vi "passTest.vi"(11 "IA state":T2={"our_robots"=[], "enemy_robots"=[], "balls"=[], "geometry"={"line_width"=0, "field_length"=0, "field_width"=0, "boundary_width"=0, "referee_width"=0, "goal_width"=0, "goal_depth"=0, "goal_wall_width"=0, "center_circle_radius"=0, "defense_radius"=0, "defense_stretch"=0, "free_kick_from_defense_dist"=0, "penalty_spot_from_field_line_dist"=0, "penalty_line_from_spot_dist"=0}, "IA Judge"={"stage"="", "command"="", "our_goalie_id"=0.0, "enemy_goalie_id"=0.0, "command enum"=enum."Halt", "Time"=enum."Azul"}, "Received Timestamp"=timestamp(0 s since 1904-01-01), "Events"={"Touch"=FALSE, "Ball out"=FALSE, "id touch"=0.0, "Ball out of \nVision"=FALSE, "Ball inside \nGoalie area"=FALSE, "Robot not responding"=FALSE, "Robots responding status"=[1.0, 1.0, 1.0, 1.0, 1.0, 1.0], "Enemy Ball \nPossession"=FALSE, "Pass State"=FALSE, "id end of pass"=0.0, "Kick"=FALSE, "Id ini Possession"=0.0, "Ball Possesion"=FALSE, "Id Possesion"=0.0}}) -> (0 "ID Kicker Robot":u32, 1 "Pass finished":bool=TRUE, 2 "ID Receiving Robot":dbl, 3 "Pass state":T1)   [LabVIEW 2017]
uses:
  Core/AI Input.ctl
  Core/AI Robot.ctl
  Intel/Functions Enum.ctl
  Intel/AttackerStates.ctl
  Core/AI Ball.ctl
  Core/Field Size.ctl
  Core/AI Judge.ctl
  Intel/Command Enum.ctl
  Util/Events/Events.ctl
  passTestStates.ctl
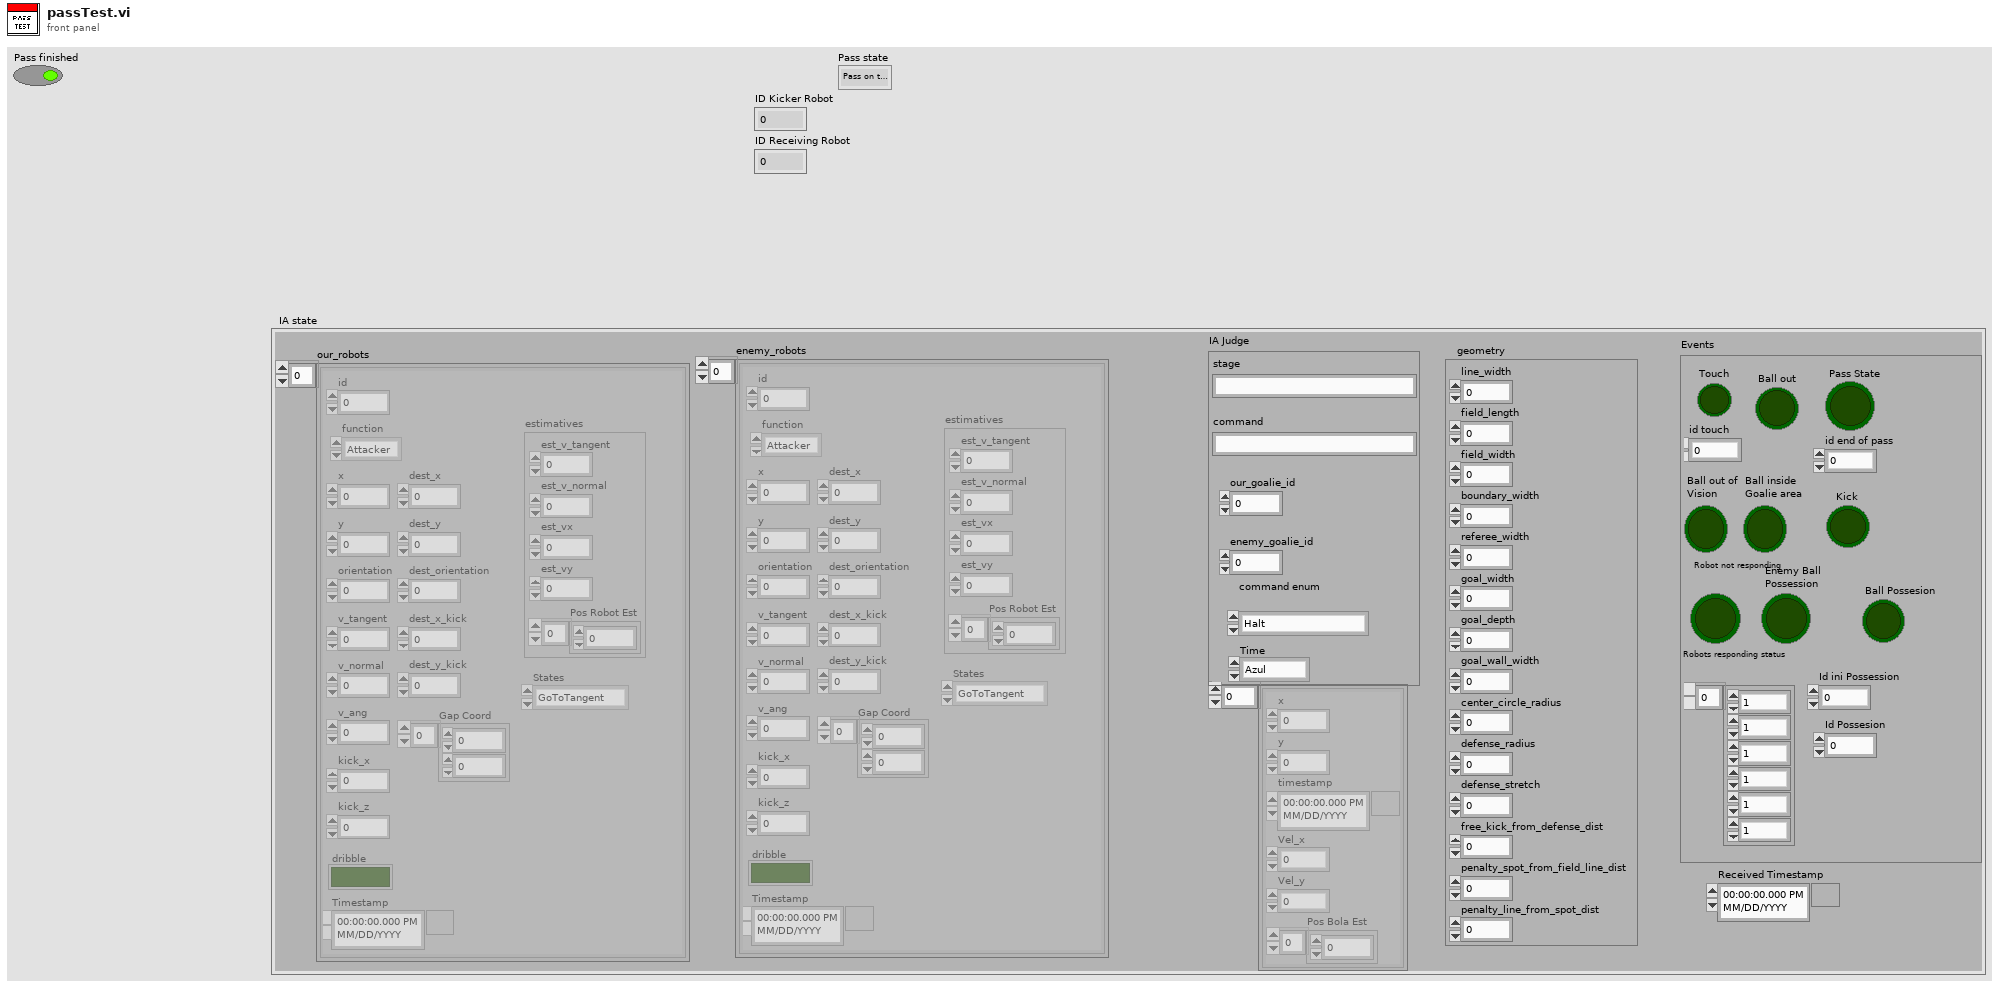
[diagram p1: front panel]
types:
  T1 = typedef "passTestStates.ctl" = enum16{"Pass on the way", "Ball stops", "Pass intercepted", "Ball out of the field", "Ball missed robot", "Need more force to pass", "Too much force", "Correct pass"}
  T2 = typedef "AI Input.ctl" = cluster{"our_robots":T3[], "enemy_robots":T3[], "balls":T6[], "geometry":T7, "IA Judge":T8, "Received Timestamp":timestamp, "Events":T10}
  T3 = typedef "AI Robot.ctl" = cluster{"id":u32, "function":T4, "x":dbl, "y":dbl, "orientation":dbl, "v_tangent":dbl, "v_normal":dbl, "v_ang":dbl, "kick_x":dbl, "kick_z":dbl, "dribble":bool, "Timestamp":timestamp, "dest_x":dbl, "dest_y":dbl, "dest_orientation":dbl, "estimatives":cluster{"est_v_tangent":dbl, "est_v_normal":dbl, "est_vx":dbl, "est_vy":dbl, "Pos Robot Est":dbl[]}, "dest_x_kick":dbl, "dest_y_kick":dbl, "Gap Coord":dbl[], "States":T5}
  T4 = typedef "Functions Enum.ctl" = enum16{"Attacker", "Goalie", "Defender", "Striker", "Goto 0", "Dummy", "Kicker", "ZigZag"}
  T5 = typedef "AttackerStates.ctl" = enum16{"Pass", "GoToTangent", "BallGetting", "GoToKick", ""}
  T6 = typedef "AI Ball.ctl" = cluster{"x":dbl, "y":dbl, "timestamp":timestamp, "Vel_x":dbl, "Vel_y":dbl, "Pos Bola Est":dbl[]}
  T7 = typedef "Field Size.ctl" = cluster{"line_width":u32, "field_length":u32, "field_width":u32, "boundary_width":u32, "referee_width":u32, "goal_width":u32, "goal_depth":u32, "goal_wall_width":u32, "center_circle_radius":u32, "defense_radius":u32, "defense_stretch":u32, "free_kick_from_defense_dist":u32, "penalty_spot_from_field_line_dist":u32, "penalty_line_from_spot_dist":u32}
  T8 = typedef "AI Judge.ctl" = cluster{"stage":string, "command":string, "our_goalie_id":dbl, "enemy_goalie_id":dbl, "command enum":T9, "Time":enum16{"Azul", "Amarelo"}}
  T9 = typedef "Command Enum.ctl" = enum16{"Halt", "Stop", "Force Start", "PKA Normal Start", "Prepare Kickoff Ally", "PKE Normal Start", "Prepare Kickoff Enemy", "Prepare Penalty Ally", "PPA Normal Start", "Prepare Penalty Enemy", "PPE Normal Start", "Direct Free Enemy", "Direct Free Ally", "Indirect Free Enemy", "Indirect Free Ally", "Timeout Enemy", "Timeout Ally", "Goal Enemy", "Goal Ally", "Ball Placement Enemy", "Ball Placement Ally", "Normal Half Time", "Extra Time Break", "Extra Half Time", "None", "Post Game"}
  T10 = typedef "Events.ctl" = cluster{"Touch":bool, "Ball out":bool, "id touch":dbl, "Ball out of \nVision":bool, "Ball inside \nGoalie area":bool, "Robot not responding":bool, "Robots responding status":dbl[], "Enemy Ball \nPossession":bool, "Pass State":bool, "id end of pass":dbl, "Kick":bool, "Id ini Possession":dbl, "Ball Possesion":bool, "Id Possesion":dbl}
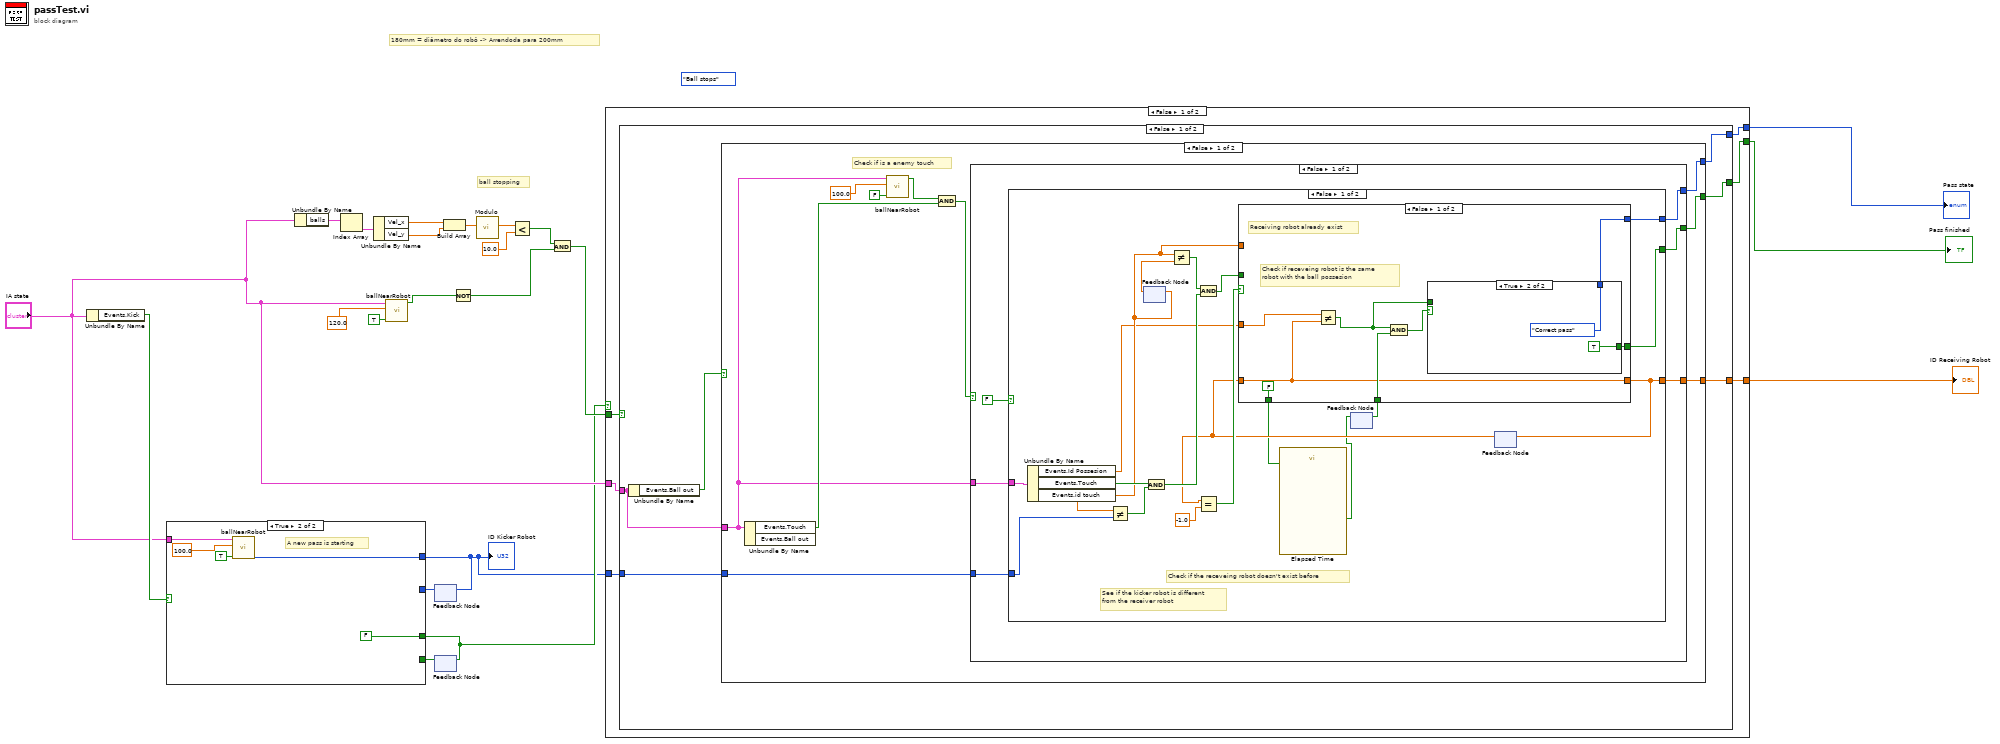
[diagram p0: block diagram]
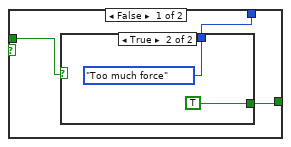
[diagram p2: hidden frame]
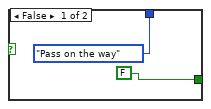
[diagram p3: hidden frame]
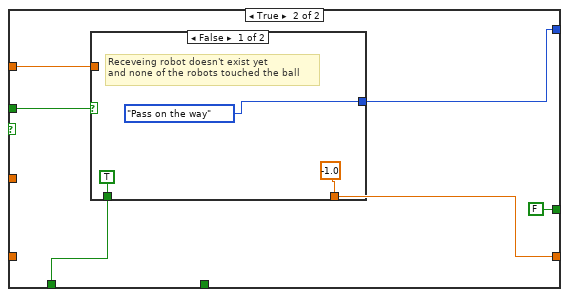
[diagram p4: hidden frame]
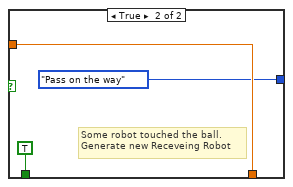
[diagram p5: hidden frame]
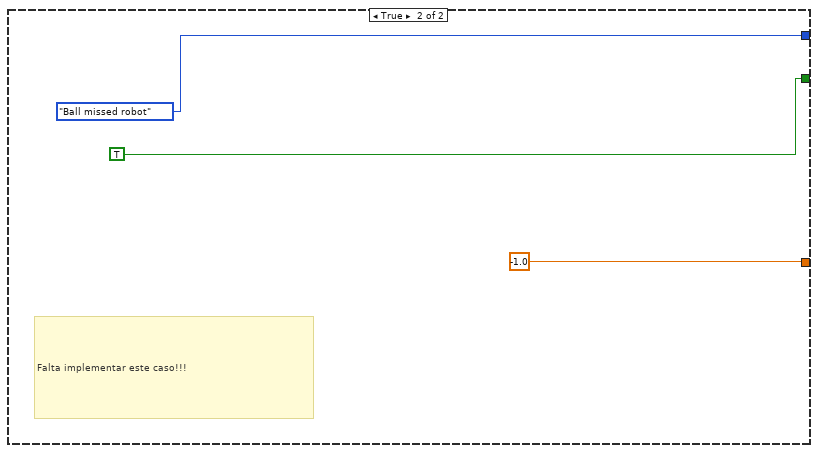
[diagram p6: hidden frame]
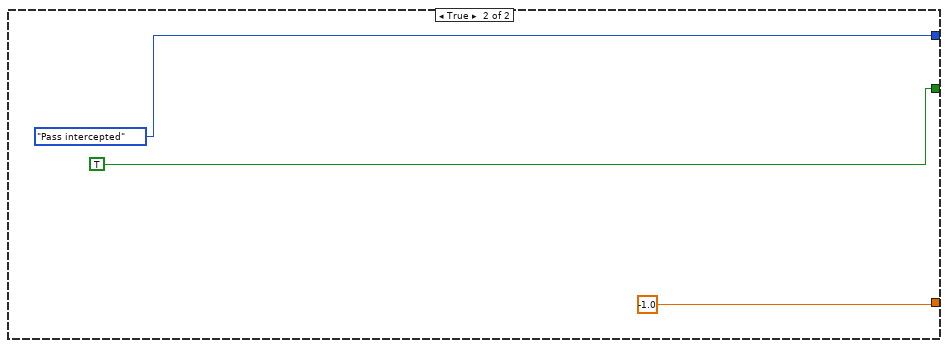
[diagram p7: hidden frame]
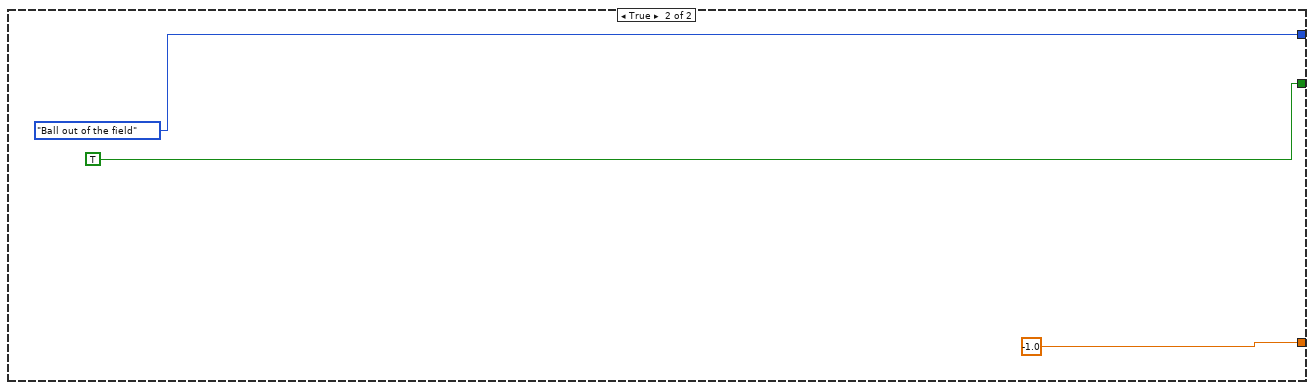
[diagram p8: hidden frame]
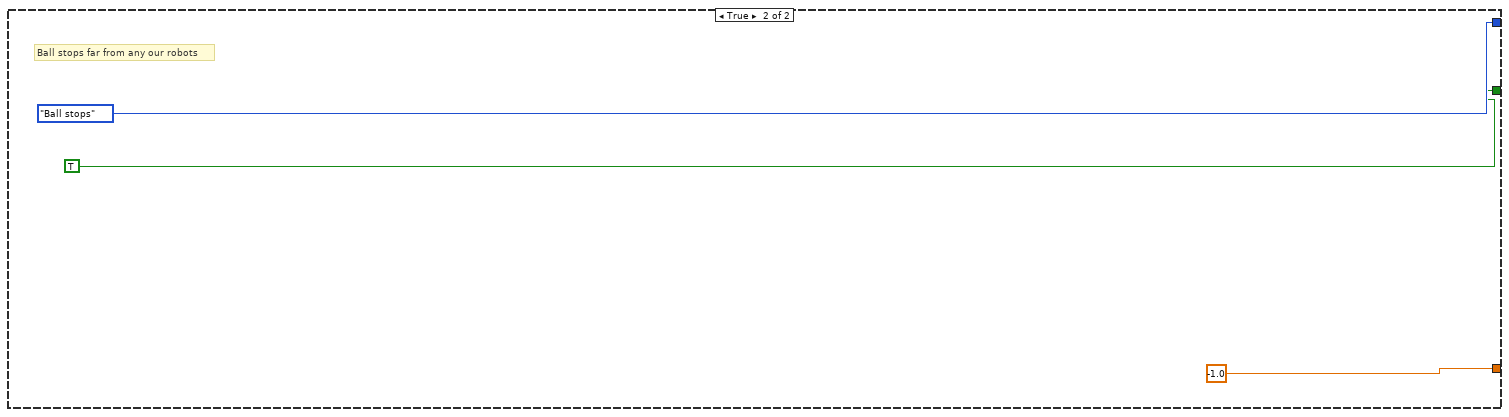
[diagram p9: hidden frame]
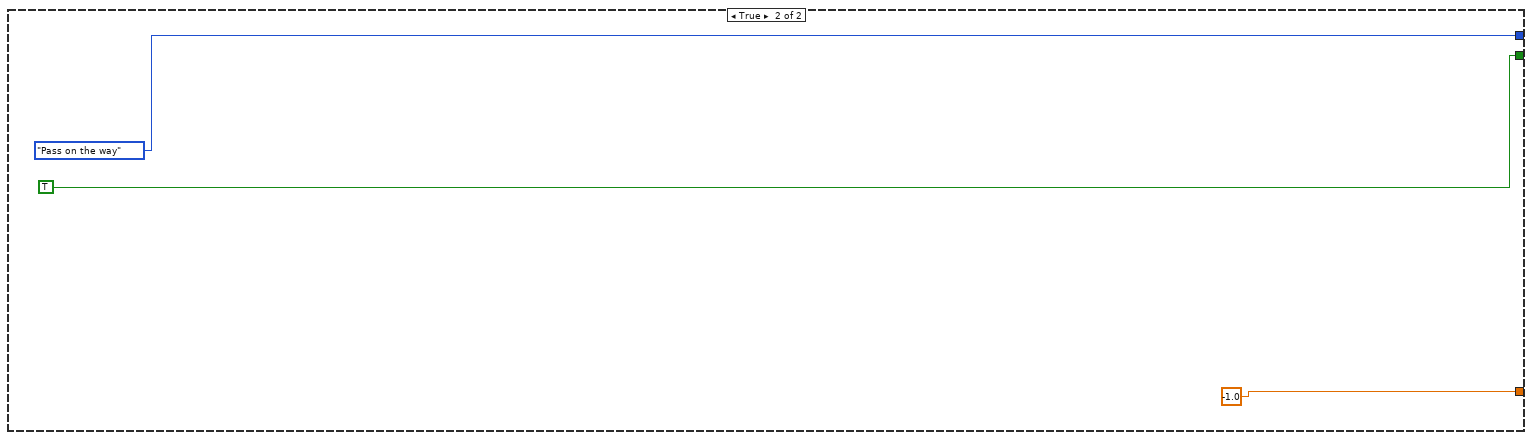
[diagram p10: hidden frame]
diagram:
  (unwired) passTestStates."Ball stops"
  # "ball stopping"
  # "180mm = diâmetro do robô -> Arrendoda para 200mm"
  n1 = Unbundle By Name("IA state") -> ("Events.Kick"=w11:bool)
  n2 = Unbundle By Name("IA state") -> ("balls"=w22:T6[])
  n3 = Index Array(array=w22) -> (element=w21:T6)  [unwired: 1 in]
  n4 = Unbundle By Name(w21) -> ("Vel_x"=w20:dbl, "Vel_y"=w19:dbl)
  n5 = call "ballNearRobot.vi"("Our robots?"=TRUE, "Distance"=120.0, "IA state"="IA state") -> ("Near to some robot"=w14:bool)  [unwired: 7 in, 1 out]
  n6 = feedback #1() -> (w9:u32)  [unwired: 1 in]
  n7 = feedback #2() -> (w8:bool)  [unwired: 1 in]
  n8 = case shown="True" w11 {
    tunnel: "IA state" -> [_ w29]
    tunnel: [w24 w26] -> w3
    tunnel: w9 -> [w24 _]
    tunnel: [w23 FALSE] -> w6
    tunnel: w8 -> [w23 _]
    frame False {
      # "A pass is already happening"
    }
    frame True {
      # "A new pass is starting"
      n9 = call "ballNearRobot.vi"("Our robots?"=TRUE, "Distance"=100.0, "IA state"=w29) -> ("ID Robot near to ball"=w26:u32)  [unwired: 7 in, 1 out]
    }
  }
  "ID Kicker Robot" <- w3
  n10 = feedback-in #1(w3) -> ()
  n11 = feedback-in #2(w6) -> ()
  n12 = Build Array(w20, w19) -> (w18:dbl[])
  n13 = Not(x=w14) -> (.not. x?=w1:bool)
  n14 = call "Modulo.vi"("2D vector"=w18) -> ("Modulo"=w17:dbl)  [unwired: 10 in]
  n15 = Less?(x=w17, y=10.0) -> (x < y?=w15:bool)
  n16 = And(x=w15, y=w1) -> (x .and. y?=w7:bool)
  n17 = case shown="False" w6 {
    tunnel: [w35 passTestStates."Pass on the way"] -> w5
    tunnel: "IA state" -> [w34 _]
    tunnel: w7 -> [w33 _]
    tunnel: [w32 TRUE] -> w4
    tunnel: w3 -> [w31 _]
    tunnel: [w30 -1.0] -> w2
    frame False {
      n18 = case shown="False" w33 {
        tunnel: [w40 passTestStates."Ball stops"] -> w35
        tunnel: w34 -> [w39 _]
        tunnel: [w38 TRUE] -> w32
        tunnel: w31 -> [w37 _]
        tunnel: [w36 -1.0] -> w30
        frame False {
          n19 = Unbundle By Name(w39) -> ("Events.Ball out"=w41:bool)
          n20 = case shown="False" w41 {
            tunnel: [w46 passTestStates."Ball out of the field"] -> w40
            tunnel: w39 -> [w44 _]
            tunnel: [w45 TRUE] -> w38
            tunnel: w37 -> [w43 _]
            tunnel: [w42 -1.0] -> w36
            frame False {
              # "Check if is a enemy touch"
              n21 = Unbundle By Name(w44) -> ("Events.Touch"=w50:bool)  [unwired: 1 out]
              n22 = call "ballNearRobot.vi"("Our robots?"=FALSE, "Distance"=100.0, "IA state"=w44) -> ("Near to some robot"=w49:bool)  [unwired: 7 in, 1 out]
              n23 = And(x=w49, y=w50) -> (x .and. y?=w47:bool)
              n24 = case shown="False" w47 {
                tunnel: [w56 passTestStates."Pass intercepted"] -> w46
                tunnel: [w55 TRUE] -> w45
                tunnel: w44 -> [w54 _]
                tunnel: w43 -> [w53 _]
                tunnel: [w52 -1.0] -> w42
                frame False {
                  n25 = case shown="False" FALSE {
                    tunnel: [w59 passTestStates."Ball missed robot"] -> w56
                    tunnel: [w58 TRUE] -> w55
                    tunnel: w54 -> [w76 _]
                    tunnel: w53 -> [w74 _]
                    tunnel: [w68 -1.0] -> w52
                    frame False {
                      # "Check if the receveing robot doesn't exist before"
                      # "See if the kicker robot is different\nfrom the receiver robot"
                      n26 = Unbundle By Name(w76) -> ("Events.Id Possesion"=w62:dbl, "Events.Touch"=w75:bool, "Events.id touch"=w70:dbl)
                      n27 = Not Equal?(x=w70, y=w74) -> (x != y?=w71:bool)
                      n28 = feedback-in #3(w70) -> ()
                      n29 = feedback #3() -> (w73:dbl)  [unwired: 1 in]
                      n30 = And(x=w75, y=w71) -> (x .and. y?=w69:bool)
                      n31 = Not Equal?(x=w70, y=w73) -> (x != y?=w72:bool)
                      n32 = And(x=w72, y=w69) -> (x .and. y?=w66:bool)
                      n33 = feedback #4() -> (w60:bool)  [unwired: 1 in]
                      n34 = feedback #5() -> (w64:dbl)  [unwired: 1 in]
                      n35 = Equal?(x=w64, y=-1.0) -> (x = y?=w65:bool)
                      n36 = case shown="False" w65 {
                        tunnel: [w77 w99] -> w68
                        tunnel: w70 -> [_ w98]
                        tunnel: w66 -> [_ w97]
                        tunnel: w64 -> [w77 _]
                        tunnel: [FALSE w96] -> w63
                        tunnel: w62 -> [w84 _]
                        tunnel: w60 -> [w82 _]
                        tunnel: [w80 w94] -> w59
                        tunnel: [w79 FALSE] -> w58
                        frame False {
                          # "Check if receveing robot is the same\nrobot with the ball possesion"
                          # "Receiving robot already exist"
                          n37 = Not Equal?(x=w84, y=w77) -> (x != y?=w78:bool)
                          n38 = And(x=w78, y=w82) -> (x .and. y?=w81:bool)
                          n39 = case shown="True" w81 {
                            tunnel: [w86 passTestStates."Correct pass"] -> w80
                            tunnel: [w85 TRUE] -> w79
                            tunnel: w78 -> [w87 _]
                            frame False {
                              n40 = case shown="True" w87 {
                                tunnel: [passTestStates."Pass on the way" passTestStates."Too much force"] -> w86
                                tunnel: [FALSE TRUE] -> w85
                                frame False {
                                }
                                frame True {
                                }
                              }
                            }
                            frame True {
                            }
                          }
                        }
                        frame True {
                          n41 = case shown="False" w97 {
                            tunnel: [-1.0 ("id touch") w105] -> w99
                            tunnel: w98 -> [_ w105]
                            tunnel: [TRUE TRUE] -> w96
                            tunnel: [passTestStates."Pass on the way" passTestStates."Pass on the way"] -> w94
                            frame False {
                              # "Receveing robot doesn't exist yet\nand none of the robots touched the ball"
                            }
                            frame True {
                              # "Some robot touched the ball.\nGenerate new Receveing Robot"
                            }
                          }
                        }
                      }
                      n42 = call "Elapsed Time"("Reset"=w63) -> ("Time has Elapsed"=w61:bool)  [unwired: 11 in, 7 out]
                      n43 = feedback-in #4(w61) -> ()
                      n44 = feedback-in #5(w68) -> ()
                    }
                    frame True {
                      # "Falta implementar este caso!!!"
                    }
                  }
                }
                frame True {
                }
              }
            }
            frame True {
            }
          }
        }
        frame True {
          # "Ball stops far from any our robots"
        }
      }
    }
    frame True {
    }
  }
  "Pass finished" <- w4
  "Pass state" <- w5
  "ID Receiving Robot" <- w2
